vi "ReadMeasurements.vi"(0 "UDP Network Connection in":refnum<k16>, 1 "Community Name":string, 2 "IP Address of SNMP Device":string, 3 "RoomAlert in":refnum<class "RoomAlert.lvclass">, 5 "Measurements To Read Array":u16[](array[numeric]), 7 "OID Numbers":string[](array[string]), 9 "Instrument Model ID":string, 11 "error in (no error)":errorcluster, 12 "Timeout(ms)":i32, 13 "Filter OID Numbers? (T)":bool=TRUE) -> (4 "UDP Network Connection out":refnum<k16>, 6 "RoomAlert Out":refnum<class "RoomAlert.lvclass">, 10 "SNMPDataAsStrings":string[][](array[string]), 15 "error out":errorcluster)   [LabVIEW 2018, in "SensorPlugins.lvlib" / "RoomAlert.lvclass"]
doc: "Reads measurements from all the sensors."
uses:
  RoomAlert.lvclass
  <vilib>/Utility/error.llb/Error Cluster From Error Code.vi
  <vilib>/ErrorRing/Error Ring.xnode
panel:
  out "OID Numbers 2":string[](array[string])
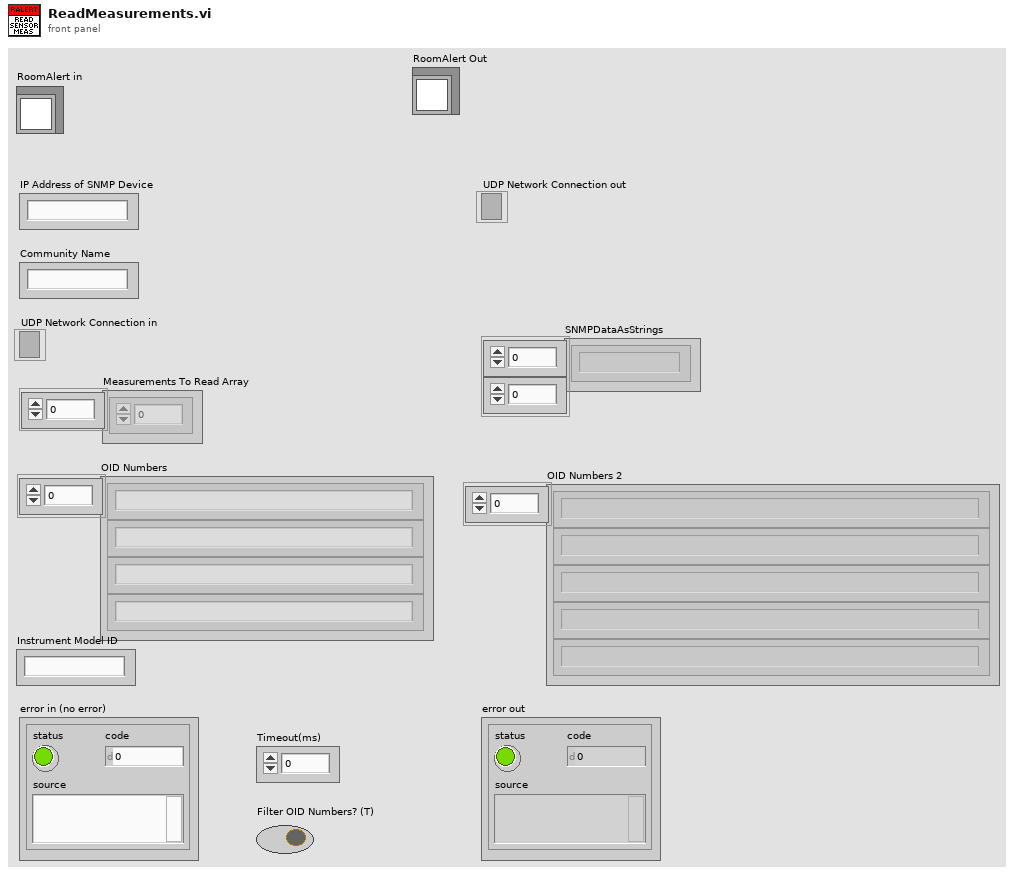
[diagram p1: front panel]
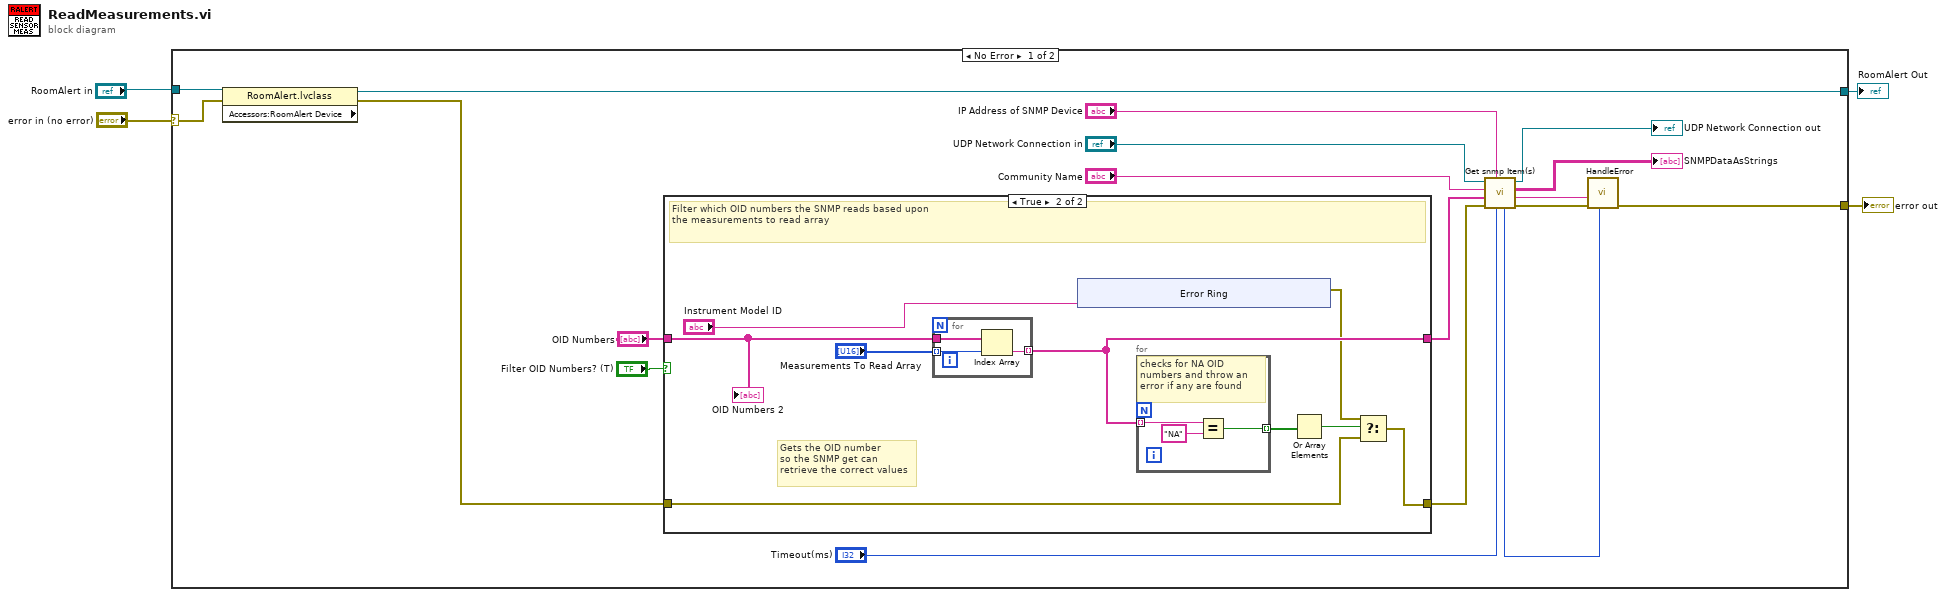
[diagram p0: block diagram]
diagram:
  n1 = case shown="No Error" "error in (no error)" {
    selector: "error in (no error)" -> [w7 w48]
    tunnel: [w22 w48] -> w4
    tunnel: "RoomAlert in" -> [w8 w47]
    tunnel: [w5 w47] -> w1
    frame No Error {
      n2 = property class="RoomAlert.lvclass" props=["Accessors:RoomAlert Device"](reference=w8, error in=w7) -> (reference out=w5:refnum<class "RoomAlert.lvclass">, error out=w6:errorcluster)  [unwired: 1 out]
      n3 = case shown="True" "Filter OID Numbers? (T)" {
        tunnel: [w24 w31] -> w13
        tunnel: "OID Numbers" -> [w24 w32]
        tunnel: w6 -> [w23 w28]
        tunnel: [w23 w27] -> w9
        frame False {
          # "Just pass through the OID number without filtering."
        }
        frame True {
          # "Gets the OID number\nso the SNMP get can \nretrieve the correct values"
          # "Filter which OID numbers the SNMP reads based upon \nthe measurements to read array"
          n4 = for {
            tunnel: "Measurements To Read Array" -> [w45] mode=indexing
            tunnel: w32 -> [w46]
            tunnel: [w44] -> w31 mode=indexing
            n5 = Index Array(array=w46, index=w45) -> (element=w44:string)
          }
          n6 = xnode "Error Ring"("parameter 0"="Instrument Model ID") -> ("error out"=w26:errorcluster)
          n7 = for {
            tunnel: w31 -> [w43] mode=indexing
            tunnel: [w41] -> w30 mode=indexing
            # "checks for NA OID \nnumbers and throw an\nerror if any are found"
            n8 = Equal?(x=w43, y="NA") -> (x = y?=w41:bool)
          }
          n9 = Or Array Elements(Boolean array=w30) -> (logical OR=w29:bool)
          n10 = Select(t=w26, s=w29, f=w28) -> (s? t:f=w27:errorcluster)
          "OID Numbers 2" <- w32
        }
      }
      n11 = call "Get snmp Item(s).vi"("timeout ms (25000)"="Timeout(ms)", "IP Address of SNMP Device"="IP Address of SNMP Device", "error in (no error)"=w9, "OID ARRAY"=w13, "Community Name"="Community Name", "connection ID in"="UDP Network Connection in") -> ("error out"=w14:errorcluster, "error-string"=w16:string, "SnmpDataAsStrings"=→"SNMPDataAsStrings":string[][], "connection ID out"=→"UDP Network Connection out":refnum<k16>, "error-status"=w12:u8)  [unwired: 1 in]
      n12 = call "HandleError.vi"("error-status"=w12, "Error In"=w14, "Error String"=w16) -> ("Error Out"=w22:errorcluster)  [unwired: 8 in]
    }
    frame Error {
    }
  }
  "error out" <- w4
  "RoomAlert Out" <- w1
